vi "Loop_Camera.vi"(10 "Camera Occurance":refnum<k4>) -> ()   [LabVIEW 2017, in "VisionHW.lvlib"]
uses:
  VisionHW.lvlib
  TypeDef/CLUST_Targeting Data.ctl
  TypeDef/CLUST_Cube Data.ctl
  TypeDef/CLUST_Road Navigation Data.ctl
  TypeDef/ENUM_Vision_Commands.ctl
  <vilib>/Rock Robotics/WPI/SerialPort/WPI_SerialPortRef.ctl
  _SHARE ALL/Global Share All/Global_STOP.vi
  Globals/Global_Vision_Data.vi
panel:
  in  "Calc":bool
  out "Targeting Data":T1
  out "Target Data":string
  in  "Vision Command":string
  out "Cycle Time (S)":dbl format="%.3g"
  in  "Target Time(ms)":u32=20
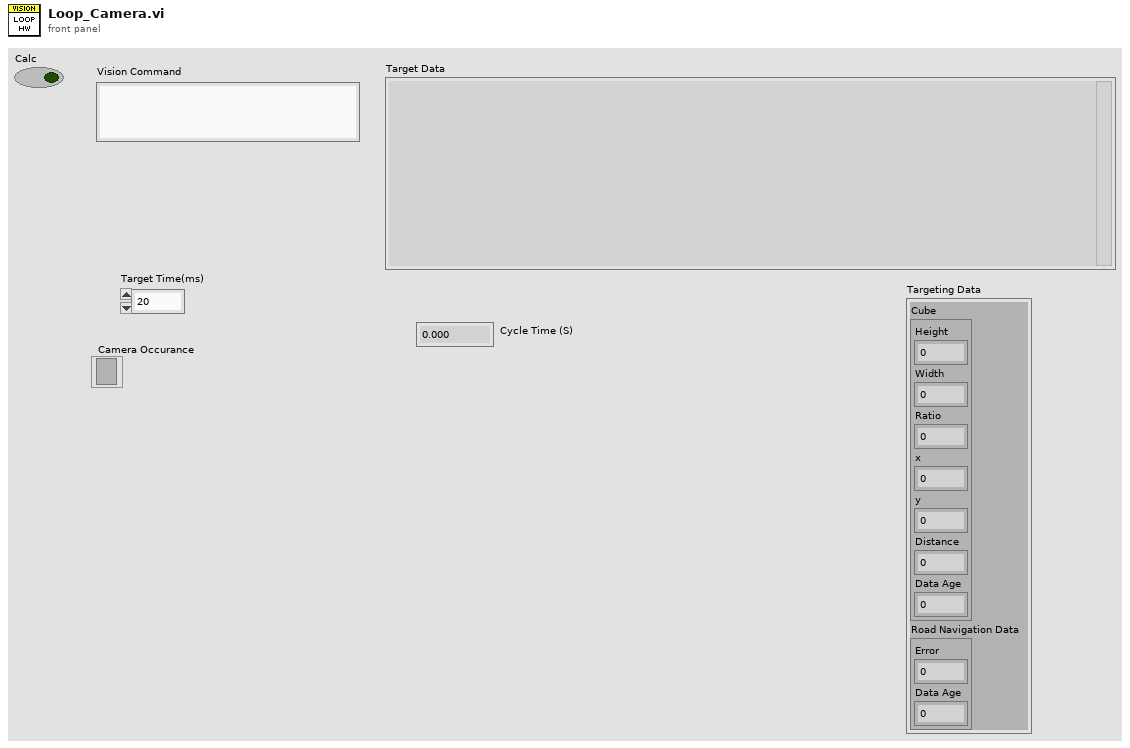
[diagram p1: front panel]
types:
  T1 = typedef "VisionHW.lvlib/CLUST_Targeting Data.ctl" = cluster{"Cube ":T2, "Road Navigation Data":T3}
  T2 = typedef "VisionHW.lvlib/CLUST_Cube Data.ctl" = cluster{"Height":dbl, "Width":dbl, "Ratio":dbl, "x":i32, "y":i32, "Distance ":i32, "Data Age":dbl}
  T3 = typedef "VisionHW.lvlib/CLUST_Road Navigation Data.ctl" = cluster{"Error":i32, "Data Age":dbl}
  T4 = typedef "WPI_SerialPortRef.ctl" = cluster{"DevStatus":errorcluster, "Serial Port Name":refnum<visa-resource-name>}
  T5 = typedef "ENUM_Vision_Commands.ctl" = enum16{"Init", "NoOp", "ResetCamera", "VideoOn", "VideoOff", "CubeDetection", "RoadNavigation"}
  T6 = cluster{"SerialRefOut":T4, " Log Output":string, "CMD":T5, "Target Time(ms)":u32, "Current Time":timestamp, "Previous Time":timestamp, "Cycle Time (S)":dbl, "Targeting Data":T1}
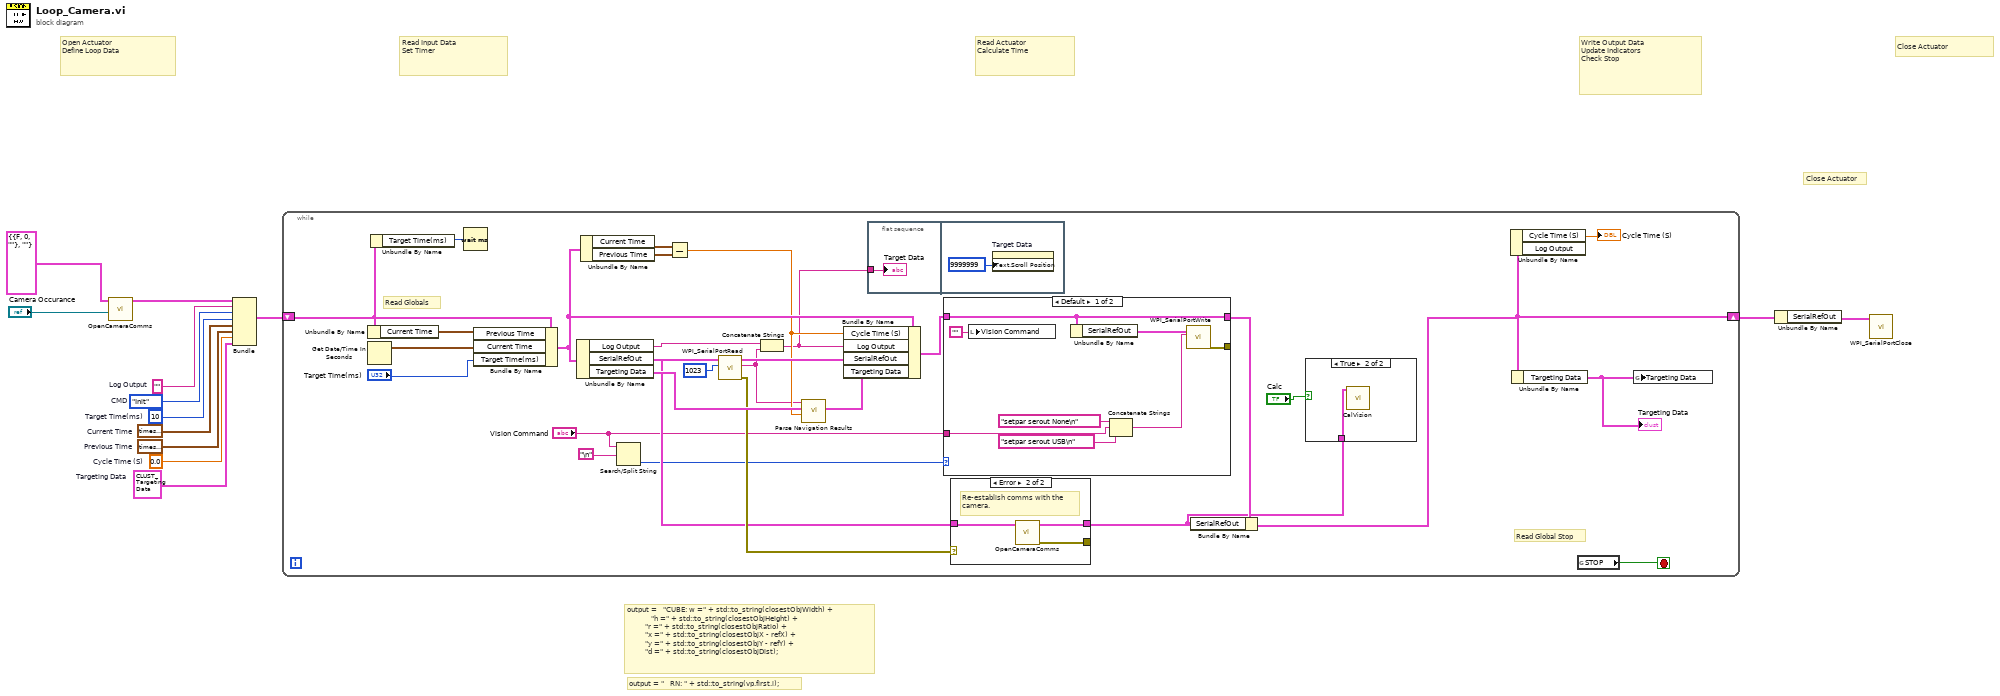
[diagram p0: block diagram]
diagram:
  w5 = T1 {"Cube "={"Height"=0.0, "Width"=0.0, "Ratio"=0.0, "x"=0, "y"=0, "Distance "=0, "Data Age"=0.0}, "Road Navigation Data"={"Error"=0, "Data Age"=0.0}}  # Targeting Data
  w8 = ENUM_Vision_Commands."Init"  # CMD
  w6 = 0.0  # Cycle Time (S)
  w13 = timestamp(0 s since 1904-01-01)  # Previous Time
  w12 = timestamp(0 s since 1904-01-01)  # Current Time
  w11 = u32 10  # Target Time(ms)
  w10 = ""  # Log Output
  # "output = \"   RN: \" + std::to_string(vp.first.i);"
  # "output =   \"CUBE: w =\" + std::to_string(closestObjWidth) +\n\t\t   \t\t\t\t\t  \"h =\" + std::to_string(closestObjHeight) +\n\t\t\t\t\t\t\t  \"r =\" + std::to_string(closestObjRatio) +\n\t\t\t\t\t\t\t  \"x =\" + std::to_string(closestObjX - refX) +\n\t\t\t\t\t\t\t  \"y =\" + std::to_string(closestObjY - refY) +\n\t\t\t\t\t\t\t  \"d =\" + std::to_string(closestObjDist);"
  # "Close Actuator"
  # "Write Output Data\nUpdate Indicators\nCheck Stop"
  # "Read Actuator\nCalculate Time"
  # "Read Input Data\nSet Timer"
  # "Open Actuator\nDefine Loop Data"
  # "Close Actuator"
  n1 = call "OpenCameraComms.vi"("Camera Occurance"="Camera Occurance", "SerialPortRef"=T4 {"DevStatus"={"status"=FALSE, "code"=0, "source"=""}, "Serial Port Name"=""}) -> ("SerialRefOut"=w7:T4)  [unwired: 8 in, 1 out]
  n2 = Bundle("SerialRefOut"=w7, "Log Output"=w10, "CMD"=w8, "Target Time(ms)"=w11, "Current Time"=w12, "Previous Time"=w13, "Cycle Time (S)"=w6, "Targeting Data"=w5) -> (w4:T6)  [unwired: 1 in]
  n3 = while {
    shift-right: [w25] -> w9
    shift-left: w4 -> [w33]
    stop <- w42 stop-if-true
    # "Read Globals"
    # "Read Global Stop"
    n4 = Unbundle By Name(w33) -> ("Current Time"=w40:timestamp)
    n5 = Get Date/Time In Seconds() -> (seconds since 1Jan1904=w41:timestamp)
    n6 = Unbundle By Name(w33) -> ("Target Time(ms)"=w35:u32)
    n7 = Wait (ms)(milliseconds to wait=w35) -> ()  [unwired: 1 out]
    n8 = Bundle By Name(cluster=w33, "Previous Time"=w40, "Current Time"=w41, "Target Time(ms)"="Target Time(ms)") -> (w36:T6)
    n9 = Unbundle By Name(w36) -> ("Log Output"=w23:string, "SerialRefOut"=w31:T4, "Targeting Data"=w30:T1)
    n10 = Unbundle By Name(w36) -> ("Current Time"=w39:timestamp, "Previous Time"=w38:timestamp)
    n11 = Search/Split String(string="Vision Command", search string/char (-)="\n") -> (offset of match=w18:i32)  [unwired: 1 in, 2 out]
    n12 = Subtract(x=w39, y=w38) -> (x-y=w22:dbl)
    n13 = call <vilib>:"WPI_SerialPortRead.vi"("Num Bytes to Read"=u32 1023 ("byte count"), "SerialPortRef"=w31) -> ("error out"=w27:errorcluster, "Buffer"=w20:string, "SerialPortRef"=w24:T4)  [unwired: 7 in]
    n14 = Concatenate Strings(w23, w20) -> (w21:string)
    n15 = call "Parse Navigation Results.vi"("Cycle Time"=w22, "Targeting Data In"=w30, "Target Data"=w20) -> ("Targeting Data Out"=w29:T1)  [unwired: 8 in]
    n16 = Bundle By Name(cluster=w36, "Cycle Time (S)"=w22, "Log Output"=w21, "SerialRefOut"=w24, "Targeting Data"=w29) -> (w16:T6)
    n17 = flat-sequence {
      tunnel: w21 -> [w48]
      frame #0 {
        "Target Data" <- w48
      }
      frame #1 {
        n18 = property on="Target Data" class="Str"("Text.Scroll Position"=u32 9999999) -> ()  [unwired: 2 in, 2 out]
      }
    }
    n19 = case shown="Default" w18 {
      tunnel: w16 -> [w57 w58]
      tunnel: [w57 w58] -> w26
      tunnel: "Vision Command" -> [w54 _]
      tunnel: [w50 _] -> _
      frame Default {
        n20 = local write "Vision Command"("") -> ()
        n21 = Unbundle By Name(w57) -> ("SerialRefOut"=w56:T4)
        n22 = Concatenate Strings("setpar serout None\n" ("string"), w54, "setpar serout USB\n" ("string")) -> (w52:string)
        n23 = call <vilib>:"WPI_SerialPortWrite.vi"("Buffer"=w52, "SerialPortRef"=w56) -> ("error out"=w50:errorcluster)  [unwired: 7 in, 2 out]
      }
      frame ..0 {
      }
    }
    n24 = case shown="Error" w27 {
      tunnel: [_ w47] -> _
      tunnel: [w44 w46] -> w15
      tunnel: w24 -> [w44 w45]
      frame No Error {
      }
      frame Error {
        # "Re-establish comms with the\ncamera."
        n25 = call "OpenCameraComms.vi"("SerialPortRef"=w45) -> ("error out"=w47:errorcluster, "SerialRefOut"=w46:T4)  [unwired: 9 in]
      }
    }
    n26 = Bundle By Name(cluster=w26, "SerialRefOut"=w15) -> (w25:T6)
    n27 = case shown="True" "Calc" {
      tunnel: w15 -> [_ w43]
      frame False {
      }
      frame True {
        n28 = call "CalVision.vi"("SerialPortIn"=w43) -> ()  [unwired: 9 in, 1 out]
      }
    }
    n29 = Unbundle By Name(w25) -> ("Cycle Time (S)"=→"Cycle Time (S)":dbl)  [unwired: 1 out]
    n30 = Unbundle By Name(w25) -> ("Targeting Data"=w28:T1)
    "Targeting Data" <- w28
    n31 = global read "Global_STOP.vi" "STOP"() -> (w42:bool)
    n32 = global write "Global_Vision_Data.vi" "Targeting Data"(w28) -> ()
  }
  n33 = Unbundle By Name(w9) -> ("SerialRefOut"=w3:T4)
  n34 = call <vilib>:"WPI_SerialPortClose.vi"("SerialPortRef"=w3) -> ()  [unwired: 10 in, 1 out]
